vi "界面UI.vi"() -> ()   [LabVIEW 2016, in "德润超标留样.lvlib"]
uses:
  <vilib>/Utility/miscctls.llb/LVPointTypeDef.ctl
panel:
  out "超标留样运行状态":T1(xcontrol)
  in  "外控留样设置":bool
  in  "外控留样读取":bool
  in  "串口重开":bool
  in  "读取选择":string(combo)
  in  "超标留样设置":bool
  in  "超标留样读取":bool
  in  "VISA resource name":refnum<visa-resource-name>="COM10" caption="VISA资源名称"
  in  "写入缓冲区":string
  in  "采样模式":enum16{"定时留样", "时间等比", "同步留样", "外控留样", "超标留样"}(ring)
  in  "采样启动":bool
  in  "切换停止":bool
  in  "切换运行":bool
  in  "时间校准":bool
  out "仪器状态":T1 {"仪器时间" format="%<%Y/%m/%d %H:%M:%S>T"; "门状态" items=["关闭", "打开"]; "采样模式" items=["定时留样"=1, "时间等比"=2, "同步留样"=3, "外控留样"=4, "超标留样"=5]; "工作进程" items=["停止中"=0, "启动延时"=1, "外置泵延时"=2, "管路润洗"=3, "管存"=4, "留样"=5, "出水管路排空"=6, "采水管路排空"=7, "待机"=13]; "工作状态" items=["停止", "运行", "系统初始化"]}
  out "读取缓冲区":string
  out "source":string
  out "通讯":bool
  # "德润超标留样"
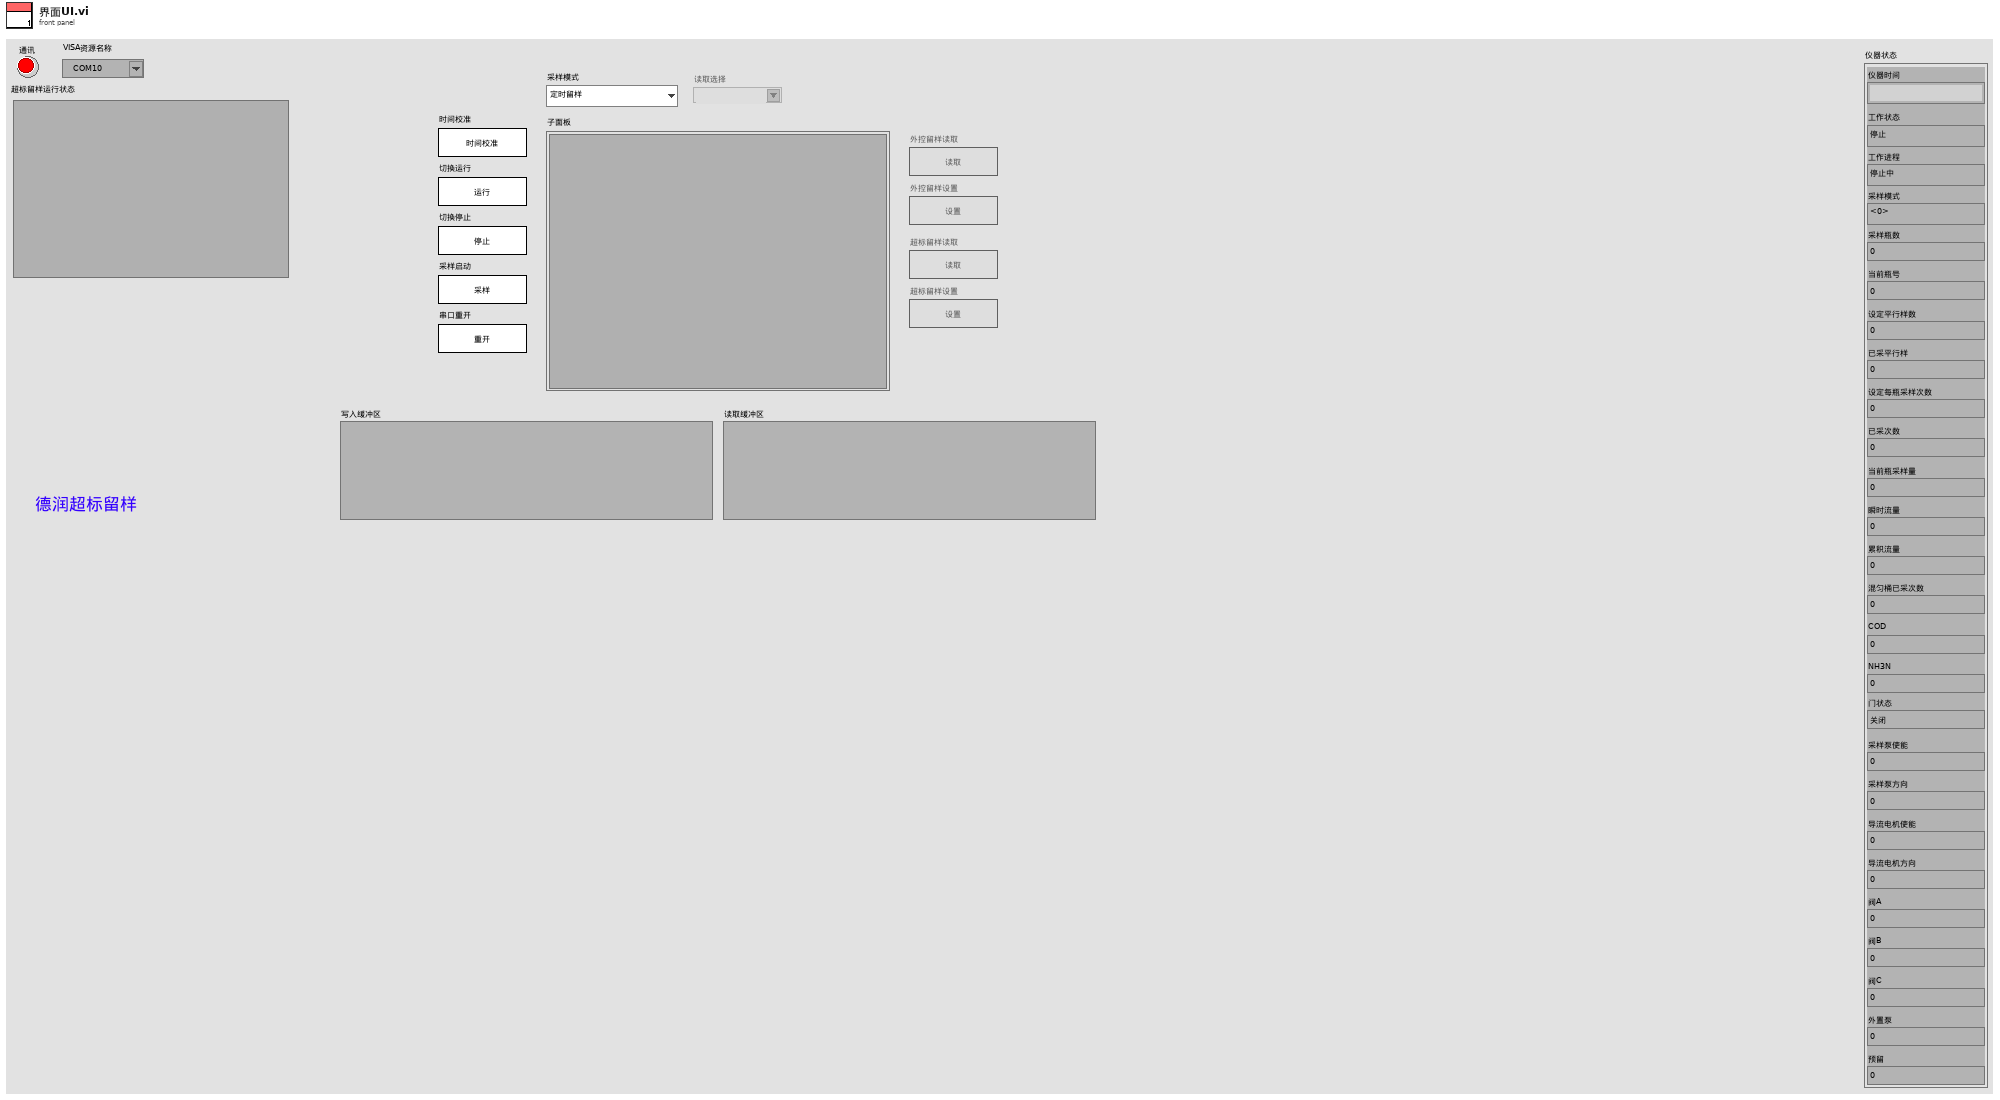
[diagram p1: front panel]
types:
  T1 = cluster{"仪器时间":timestamp, "工作状态":u16, "工作进程":u16, "采样模式":u16, "采样瓶数":dbl, "当前瓶号":dbl, "设定平行样数":dbl, "已采平行样":dbl, "设定每瓶采样次数":dbl, "已采次数":dbl, "当前瓶采样量":dbl, "瞬时流量":dbl, "累积流量":dbl, "混匀桶已采次数":dbl, "COD":dbl, "NH3N":dbl, "门状态":u16, "采样泵使能":dbl, "采样泵方向":dbl, "导流电机使能":dbl, "导流电机方向":dbl, "阀A":dbl, "阀B":dbl, "阀C":dbl, "外置泵":dbl, "预留":dbl}
  T2 = typedef "LVPointTypeDef.ctl" = cluster{"Horizontal":i16, "Vertical":i16}
  T3 = enum32{"Bad", "Idle", "Run top level", "Running"}
  T4 = cluster{"当前瓶号：":dbl, "平行样：":dbl, "留样瓶数：":dbl, "每瓶次数：":dbl, "每次留样：":dbl}
  T5 = cluster{"当前瓶号：":dbl, "平行样：":dbl, "留样瓶数：":dbl, "每瓶次数：":dbl, "每次留样：":dbl, "时间间隔：":dbl, "COD联机：":u16, "氨氮联机：":u16, "4mA浓度：":dbl, "20mA浓度：":dbl, "超标浓度：":dbl, "4mA浓度：":dbl, "20mA浓度:":dbl, "超标浓度：":dbl}
  T6 = enum8{"Enabled", "Disabled", "Disabled and Grayed Out"}
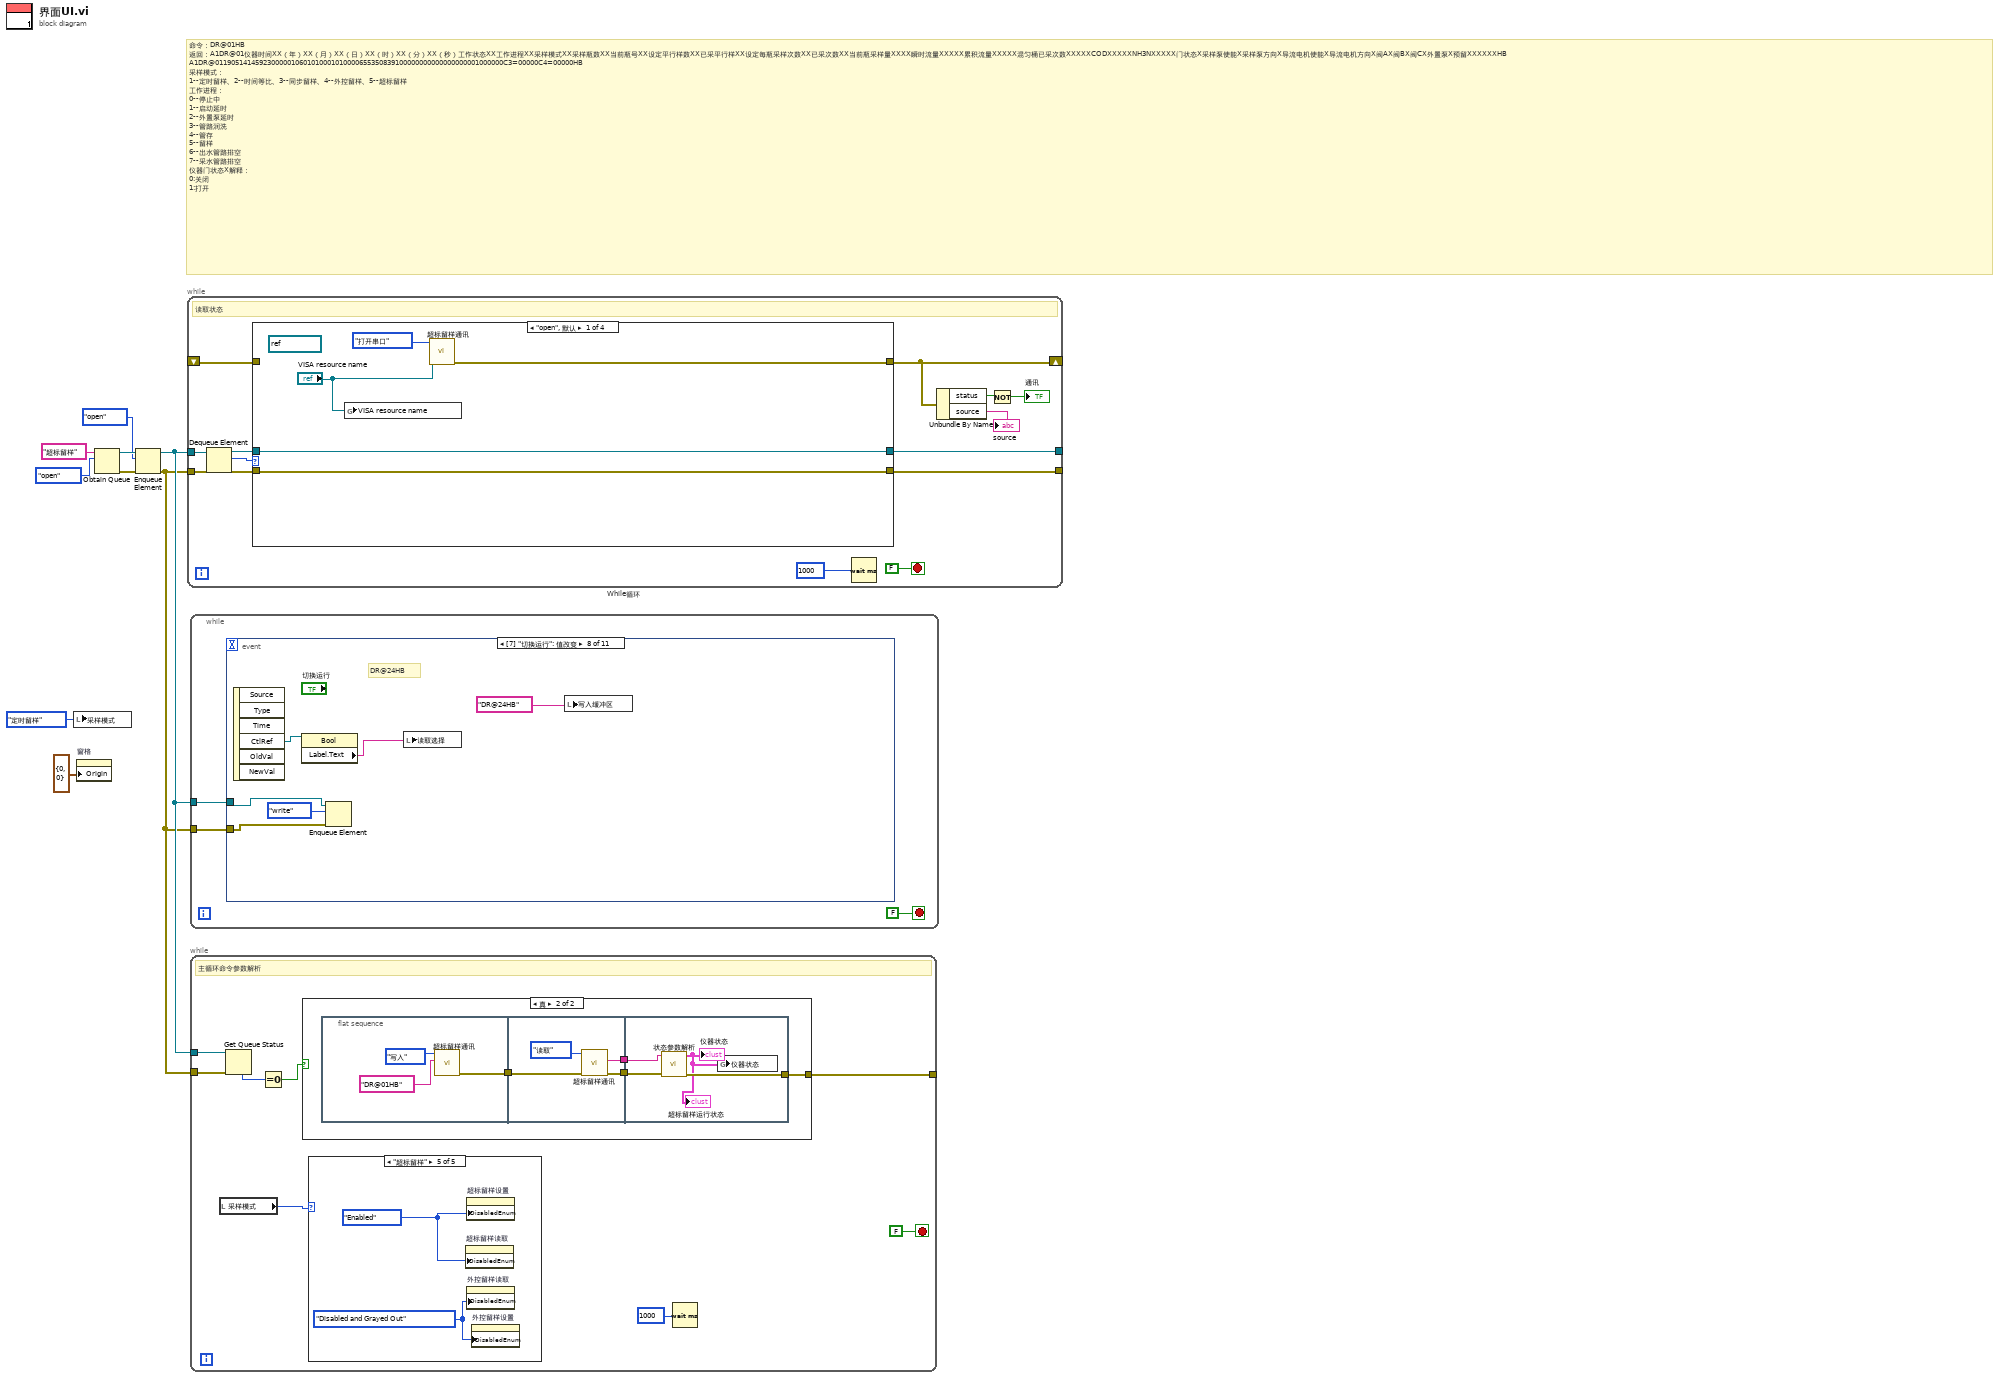
[diagram p0: block diagram]
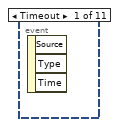
[diagram p2: hidden frame]
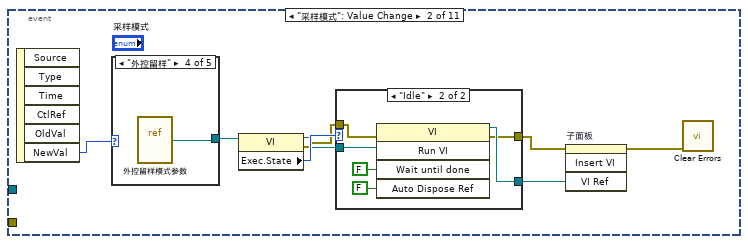
[diagram p3: hidden frame]
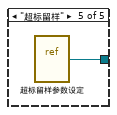
[diagram p8: hidden frame]
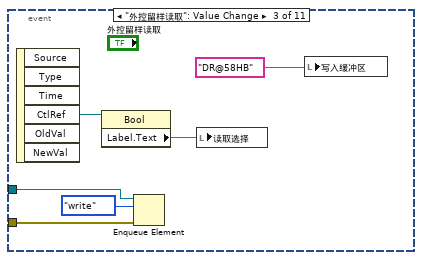
[diagram p9: hidden frame]
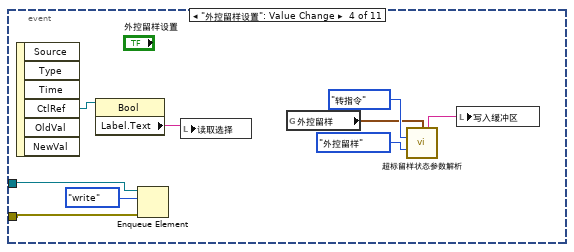
[diagram p10: hidden frame]
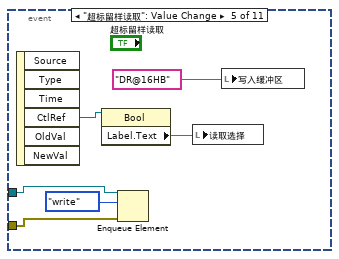
[diagram p11: hidden frame]
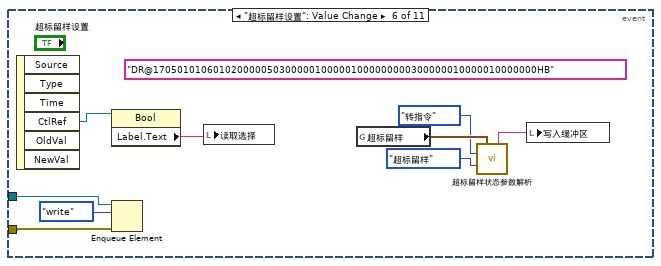
[diagram p12: hidden frame]
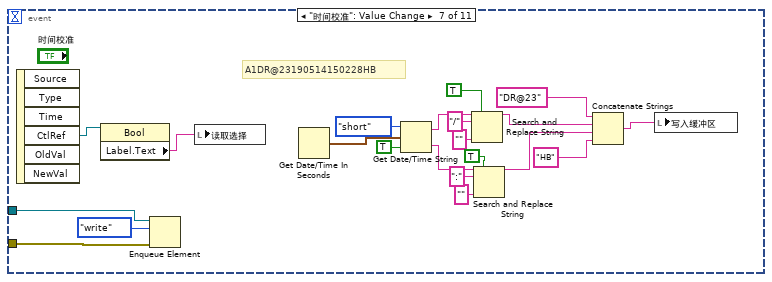
[diagram p13: hidden frame]
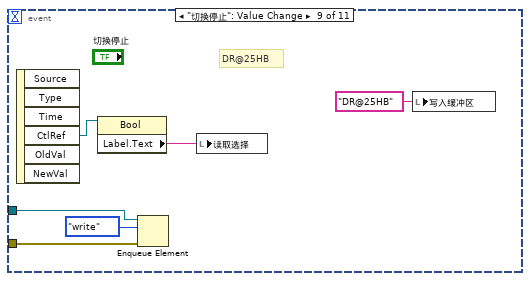
[diagram p14: hidden frame]
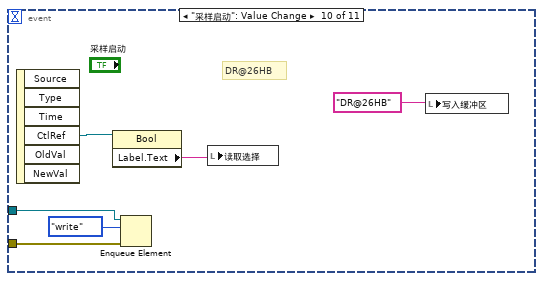
[diagram p15: hidden frame]
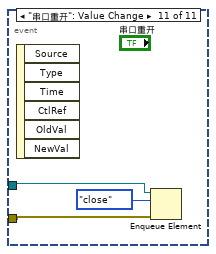
[diagram p16: hidden frame]
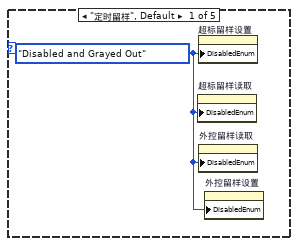
[diagram p18: hidden frame]
diagram:
  # "命令：DR@01HB\n返回：A1DR@01仪器时间XX（年）XX（月）XX（日）XX（时）XX（分）XX（秒）工作状态XX工作进程XX采样模式XX采样瓶数XX当前瓶号XX设定平行样数XX已采平行样XX设定每瓶采样次数XX已采次数XX当前瓶采样量XXXX瞬时流量XXXXX累积流量XXXXX混匀桶已采次数XXXXXCODXXXXXNH3NXXXXX门状态X采样泵使能X采样泵方向X导流电机使能X导流电机方向X阀AX阀BX阀CX外置泵X预留XXXXXXHB\nA1DR@011905141459230000010601010001010000655350839100000000000000000001000000C3=00000C4=00000HB\n采样模式：\n1--定时留样、2--时间等比、3--同步留样、4--外控留样、5--超标留样\n工作进程：\n0--停止中\n1--启动延时\n2--外置泵延时\n3--管路润洗\n4--管存\n5--留样\n6--出水管路排空\n7--采水管路排空\n仪器门状态X解释：\n0:关闭\n1:打开"
  n1 = local write "采样模式"(enum16{"定时留样", "时间等比", "同步留样", "外控留样", "超标留样"}."定时留样" ("采样模式")) -> ()
  n2 = property on="窗格" class="Pane"("Origin"=T2 {"Horizontal"=0, "Vertical"=0} ("原点")) -> ()  [unwired: 2 in, 2 out]
  n3 = Obtain Queue(name (unnamed)="超标留样" ("名称（未命名）"), element data type=enum16{"open", "read", "write", "close"}."open") -> (queue out=w7:refnum<queue>, error out=w6:errorcluster)  [unwired: 3 in, 1 out]
  n4 = Enqueue Element(queue=w7, element=enum16{"open", "read", "write", "close"}."open", error in (no error)=w6) -> (queue out=w3:refnum<queue>, error out=w2:errorcluster)  [unwired: 1 in, 1 out]
  n5 = while "While循环" {
    tunnel: w3 -> [w21]
    tunnel: w2 -> [w20]
    tunnel: [w16] -> _
    tunnel: [w15] -> _
    shift-right: [w10] -> _
    shift-left: _ -> [w14]
    stop <- FALSE stop-if-true
    # "读取状态"
    n6 = Dequeue Element(queue=w21, error in (no error)=w20) -> (queue out=w18:refnum<queue>, element=w19:enum16{"open", "read", "write", "close"}, error out=w17:errorcluster)  [unwired: 1 in, 1 out]
    n7 = case shown="\"open\", 默认" w19 {
      tunnel: [w27 w34 w57 w69] -> w10
      tunnel: w18 -> [w26 w32 w62 w68]
      tunnel: w17 -> [w25 w31 w61 w67]
      tunnel: [w26 w32 w60 w65] -> w16
      tunnel: [w25 w31 w59 w64] -> w15
      tunnel: w14 -> [_ w35 w58 w71]
      frame "open", Default {
        (unwired) refnum<visa-resource-name> "COM2" ("VISA resource name")
        n8 = global write "超标留样全局.vi" "VISA resource name"("VISA resource name") -> ()
        n9 = call "超标留样通讯.vi"("VISA resource name"="VISA resource name", "功能输入"=enum16{"打开串口", "写入", "读取", "关闭串口"}."打开串口") -> ("error out"=w27:errorcluster)  [unwired: 7 in, 2 out]
      }
      frame "read" {
        n10 = call "超标留样通讯.vi"("error in (no error)"=w35, "功能输入"=enum16{"打开串口", "写入", "读取", "关闭串口"}."读取") -> ("error out"=w34:errorcluster, "读取缓冲区"=w29:string)  [unwired: 7 in, 1 out]
        "读取缓冲区" <- w29
        n11 = case shown="\"外控留样读取\"" "读取选择" {
          tunnel: w29 -> [w36 w43 w54]
          frame "超标留样读取" {
            n12 = flat-sequence {
              tunnel: w36 -> [w39]
              frame #0 {
                n13 = call "超标留样状态参数解析.vi"("输入字符串"=w39, "解析/转指令"=enum16{"解析", "转指令"}."解析", "模式选择"=enum16{"外控留样", "超标留样"}."超标留样") -> ()  [unwired: 11 in, 2 out]
              }
              frame #1 {
                n14 = global write "超标留样全局.vi" "读取更新"(TRUE ("读取更新")) -> ()
              }
              frame #2 {
                n15 = Wait (ms)(milliseconds to wait=u32 500 ("等待时间（毫秒）")) -> ()  [unwired: 1 out]
              }
              frame #3 {
                n16 = global write "超标留样全局.vi" "读取更新"(FALSE ("读取更新")) -> ()
              }
            }
          }
          frame "外控留样读取" {
            n17 = flat-sequence {
              tunnel: w43 -> [w44]
              frame #0 {
                n18 = call "超标留样状态参数解析.vi"("输入字符串"=w44, "解析/转指令"=enum16{"解析", "转指令"}."解析", "模式选择"=enum16{"外控留样", "超标留样"}."外控留样") -> ()  [unwired: 11 in, 2 out]
              }
              frame #1 {
                n19 = global write "超标留样全局.vi" "外控留样读取更新"(TRUE ("读取更新")) -> ()
              }
              frame #2 {
                n20 = Wait (ms)(milliseconds to wait=u32 500 ("等待时间（毫秒）")) -> ()  [unwired: 1 out]
              }
              frame #3 {
                n21 = global write "超标留样全局.vi" "外控留样读取更新"(FALSE ("读取更新")) -> ()
              }
            }
          }
          frame "超标留样设置", Default {
            n22 = String Subset(string=w54, offset (0)=5 ("偏移量(0)")) -> (substring=w52:string)  [unwired: 1 in]
            n23 = Search/Split String(string=w52, search string/char (-)="HB" ("搜索字符串/字符(-)")) -> (substring before match=w50:string)  [unwired: 1 in, 2 out]
            n24 = One Button Dialog(message=w50) -> ()  [unwired: 1 in, 1 out]
          }
        }
      }
      frame "write" {
        n25 = call "超标留样通讯.vi"("error in (no error)"=w58, "写入缓冲区"="写入缓冲区", "功能输入"=enum16{"打开串口", "写入", "读取", "关闭串口"}."写入") -> ("error out"=w57:errorcluster)  [unwired: 6 in, 2 out]
        n26 = Enqueue Element(queue=w62, element=enum16{"open", "read", "write", "close"}."read" ("元素"), error in (no error)=w61) -> (queue out=w60:refnum<queue>, error out=w59:errorcluster)  [unwired: 1 in, 1 out]
      }
      frame "close" {
        n27 = call "超标留样通讯.vi"("error in (no error)"=w71, "功能输入"=enum16{"打开串口", "写入", "读取", "关闭串口"}."关闭串口") -> ("error out"=w69:errorcluster)  [unwired: 7 in, 2 out]
        n28 = Enqueue Element(queue=w68, element=enum16{"open", "read", "write", "close"}."open" ("元素"), error in (no error)=w67) -> (queue out=w65:refnum<queue>, error out=w64:errorcluster)  [unwired: 1 in, 1 out]
      }
    }
    n29 = Wait (ms)(milliseconds to wait=u32 1000 ("等待时间（毫秒）")) -> ()  [unwired: 1 out]
    n30 = Unbundle By Name(w10) -> ("status"=w11:bool, "source"=→"source":string)
    n31 = Not(x=w11) -> (.not. x?=→"通讯":bool)
  }
  n32 = while {
    tunnel: w3 -> [w73]
    tunnel: w2 -> [w72]
    stop <- FALSE stop-if-true
    n33 = event shown="[7] \"切换运行\": 值改变" {
      selector: _ -> [_ _ _ _ _ _ _ _ _ _ _]
      dyn-events: _ -> [_ _ _ _ _ _ _ _ _ _ _]
      timeout: _ -> [_ _ _ _ _ _ _ _ _ _ _]
      tunnel: w73 -> [_ _ w95 w106 w111 w121 w142 w147 w153 w159 w163]
      tunnel: w72 -> [_ _ w96 w105 w110 w120 w141 w146 w152 w158 w162]
      event Timeout {
        n34 = event-data() -> ()  [unwired: 1 in, 3 out]
      }
      event "采样模式": Value Change {
        n35 = event-data() -> ("NewVal"=w82:enum16{"定时留样", "时间等比", "同步留样", "外控留样", "超标留样"})  [unwired: 1 in, 5 out]
        n36 = case shown="\"外控留样\"" w82 {
          tunnel: [_ _ _ w91 w92] -> w81
          frame "定时留样", Default {
          }
          frame "时间等比" {
          }
          frame "同步留样" {
          }
          frame "外控留样" {
            n37 = vi-ref "外控留样模式参数.vi"() -> (w91:refnum<vi>)
          }
          frame "超标留样" {
            n38 = vi-ref "超标留样参数设定.vi"() -> (w92:refnum<vi>)
          }
        }
        n39 = property class="VI"(reference=w81) -> (reference out=w79:refnum<vi>, error out=w77:errorcluster, "Exec.State"=w80:T3)  [unwired: 1 in]
        n40 = case shown="\"Idle\"" w80 {
          tunnel: w79 -> [w84 w90]
          tunnel: [w84 w87] -> w78
          tunnel: w77 -> [w83 w86]
          tunnel: [w83 w85] -> w76
          frame "Bad", Default {
          }
          frame "Idle" {
            n41 = invoke class="VI" method="Run VI"(reference=w90, error in=w86, "Wait until done"=FALSE ("结束前等待"), "Auto Dispose Ref"=FALSE ("自动销毁引用")) -> (reference out=w87:refnum<vi>, error out=w85:errorcluster)  [unwired: 1 in, 3 out]
          }
        }
        n42 = invoke on="子面板" class="SubPnl" method="Insert VI"(error in=w76, "VI Ref"=w78) -> (error out=w75:errorcluster)  [unwired: 2 in, 3 out]
        n43 = call <vilib>:"Clear Errors.vi"("error in (no error)"=w75) -> ()  [unwired: 5 in, 2 out]
      }
      event "外控留样读取": Value Change {
        n44 = event-data() -> ("CtlRef"=w94:refnum<vi>)  [unwired: 1 in, 5 out]
        n45 = property class="Bool"(reference=w94) -> ("Label.Text"=w93:string)  [unwired: 1 in, 2 out]
        n46 = Enqueue Element(queue=w95, element=enum16{"open", "read", "write", "close"}."write" ("元素"), error in (no error)=w96) -> ()  [unwired: 1 in, 3 out]
        n47 = local write "读取选择"(w93) -> ()
        n48 = local write "写入缓冲区"("DR@58HB") -> ()
      }
      event "外控留样设置": Value Change {
        n49 = event-data() -> ("CtlRef"=w100:refnum<vi>)  [unwired: 1 in, 5 out]
        n50 = property class="Bool"(reference=w100) -> ("Label.Text"=w99:string)  [unwired: 1 in, 2 out]
        n51 = Enqueue Element(queue=w106, element=enum16{"open", "read", "write", "close"}."write" ("元素"), error in (no error)=w105) -> ()  [unwired: 1 in, 3 out]
        n52 = local write "读取选择"(w99) -> ()
        n53 = global read "超标留样全局.vi" "外控留样"() -> (w101:T4)
        n54 = call "超标留样状态参数解析.vi"("外控留样"=w101, "解析/转指令"=enum16{"解析", "转指令"}."转指令", "模式选择"=enum16{"外控留样", "超标留样"}."外控留样") -> ("输出字符串"=w102:string)  [unwired: 11 in, 1 out]
        n55 = local write "写入缓冲区"(w102) -> ()
      }
      event "超标留样读取": Value Change {
        n56 = event-data() -> ("CtlRef"=w109:refnum<vi>)  [unwired: 1 in, 5 out]
        n57 = property class="Bool"(reference=w109) -> ("Label.Text"=w108:string)  [unwired: 1 in, 2 out]
        n58 = Enqueue Element(queue=w111, element=enum16{"open", "read", "write", "close"}."write" ("元素"), error in (no error)=w110) -> ()  [unwired: 1 in, 3 out]
        n59 = local write "读取选择"(w108) -> ()
        n60 = local write "写入缓冲区"("DR@16HB") -> ()
      }
      event "超标留样设置": Value Change {
        (unwired) "DR@1705010106010200000503000001000001000000000300000010000010000000HB"
        n61 = event-data() -> ("CtlRef"=w115:refnum<vi>)  [unwired: 1 in, 5 out]
        n62 = property class="Bool"(reference=w115) -> ("Label.Text"=w114:string)  [unwired: 1 in, 2 out]
        n63 = Enqueue Element(queue=w121, element=enum16{"open", "read", "write", "close"}."write" ("元素"), error in (no error)=w120) -> ()  [unwired: 1 in, 3 out]
        n64 = local write "读取选择"(w114) -> ()
        n65 = global read "超标留样全局.vi" "超标留样"() -> (w119:T5)
        n66 = call "超标留样状态参数解析.vi"("超标留样"=w119, "解析/转指令"=enum16{"解析", "转指令"}."转指令", "模式选择"=enum16{"外控留样", "超标留样"}."超标留样") -> ("输出字符串"=w116:string)  [unwired: 11 in, 1 out]
        n67 = local write "写入缓冲区"(w116) -> ()
      }
      event "时间校准": Value Change {
        # "A1DR@23190514150228HB"
        n68 = event-data() -> ("CtlRef"=w124:refnum<vi>)  [unwired: 1 in, 5 out]
        n69 = property class="Bool"(reference=w124) -> ("Label.Text"=w123:string)  [unwired: 1 in, 2 out]
        n70 = Enqueue Element(queue=w142, element=enum16{"open", "read", "write", "close"}."write" ("元素"), error in (no error)=w141) -> ()  [unwired: 1 in, 3 out]
        n71 = local write "读取选择"(w123) -> ()
        n72 = Get Date/Time In Seconds() -> (seconds since 1Jan1904=w137:timestamp)
        n73 = Get Date/Time String(date format (0)=enum16{"short", "long", "abbreviated"}."short" ("日期格式(0)"), seconds (now)=w137, want seconds? (F)=TRUE ("需要秒？(F)")) -> (date string=w136:string, time string=w129:string)
        n74 = Search and Replace String(replace all?=TRUE ("替换全部？(F)"), input string=w136, search string="/" ("搜索字符串"), replace string="" ("替换字符串(\"\")")) -> (result string=w128:string)  [unwired: 4 in, 3 out]
        n75 = Search and Replace String(replace all?=TRUE ("替换全部？(F)"), input string=w129, search string=":" ("搜索字符串"), replace string="" ("替换字符串(\"\")")) -> (result string=w127:string)  [unwired: 4 in, 3 out]
        n76 = Concatenate Strings("DR@23" ("写入缓冲区"), w128, w127, "HB" ("写入缓冲区")) -> (w125:string)
        n77 = local write "写入缓冲区"(w125) -> ()
      }
      event "切换运行": Value Change {
        # "DR@24HB"
        n78 = event-data() -> ("CtlRef"=w145:refnum<vi>)  [unwired: 1 in, 5 out]
        n79 = property class="Bool"(reference=w145) -> ("Label.Text"=w144:string)  [unwired: 1 in, 2 out]
        n80 = Enqueue Element(queue=w147, element=enum16{"open", "read", "write", "close"}."write" ("元素"), error in (no error)=w146) -> ()  [unwired: 1 in, 3 out]
        n81 = local write "读取选择"(w144) -> ()
        n82 = local write "写入缓冲区"("DR@24HB") -> ()
      }
      event "切换停止": Value Change {
        # "DR@25HB"
        n83 = event-data() -> ("CtlRef"=w151:refnum<vi>)  [unwired: 1 in, 5 out]
        n84 = property class="Bool"(reference=w151) -> ("Label.Text"=w150:string)  [unwired: 1 in, 2 out]
        n85 = Enqueue Element(queue=w153, element=enum16{"open", "read", "write", "close"}."write" ("元素"), error in (no error)=w152) -> ()  [unwired: 1 in, 3 out]
        n86 = local write "读取选择"(w150) -> ()
        n87 = local write "写入缓冲区"("DR@25HB" ("写入缓冲区")) -> ()
      }
      event "采样启动": Value Change {
        # "DR@26HB"
        n88 = event-data() -> ("CtlRef"=w157:refnum<vi>)  [unwired: 1 in, 5 out]
        n89 = property class="Bool"(reference=w157) -> ("Label.Text"=w156:string)  [unwired: 1 in, 2 out]
        n90 = Enqueue Element(queue=w159, element=enum16{"open", "read", "write", "close"}."write" ("元素"), error in (no error)=w158) -> ()  [unwired: 1 in, 3 out]
        n91 = local write "读取选择"(w156) -> ()
        n92 = local write "写入缓冲区"("DR@26HB") -> ()
      }
      event "串口重开": Value Change {
        n93 = event-data() -> ()  [unwired: 1 in, 6 out]
        n94 = Enqueue Element(queue=w163, element=enum16{"open", "read", "write", "close"}."close" ("元素"), error in (no error)=w162) -> ()  [unwired: 1 in, 3 out]
      }
    }
  }
  n95 = while {
    tunnel: [w170] -> _
    tunnel: w3 -> [w168]
    tunnel: w2 -> [w167]
    stop <- FALSE stop-if-true
    # "主循环命令参数解析"
    n96 = local read "采样模式"() -> (w169:enum16{"定时留样", "时间等比", "同步留样", "外控留样", "超标留样"})
    n97 = Get Queue Status(queue=w168, error in (no error)=w167) -> (# elements in queue=w166:i32)  [unwired: 1 in, 7 out]
    n98 = Equal To 0?(x=w166) -> (x = 0?=w165:bool)
    n99 = case shown="真" w165 {
      tunnel: [_ w173] -> w170
      frame False {
      }
      frame True {
        n100 = flat-sequence {
          tunnel: [w177] -> w176
          tunnel: w176 -> [w182]
          tunnel: [w181] -> w175
          tunnel: [w180] -> w174
          tunnel: w175 -> [w187]
          tunnel: w174 -> [w186]
          tunnel: [w185] -> w173
          frame #0 {
            n101 = call "超标留样通讯.vi"("写入缓冲区"="DR@01HB", "功能输入"=enum16{"打开串口", "写入", "读取", "关闭串口"}."写入") -> ("error out"=w177:errorcluster)  [unwired: 7 in, 2 out]
          }
          frame #1 {
            n102 = call "超标留样通讯.vi"("error in (no error)"=w182, "功能输入"=enum16{"打开串口", "写入", "读取", "关闭串口"}."读取") -> ("error out"=w181:errorcluster, "读取缓冲区"=w180:string)  [unwired: 7 in, 1 out]
          }
          frame #2 {
            n103 = call "状态参数解析.vi"("error in (no error)"=w187, "字符串"=w186) -> ("error out"=w185:errorcluster, "簇"=w184:T1)  [unwired: 8 in]
            "仪器状态" <- w184
            "超标留样运行状态" <- w184
            n104 = global write "超标留样全局.vi" "仪器状态"(w184) -> ()
          }
        }
      }
    }
    n105 = case shown="\"超标留样\"" w169 {
      frame "定时留样", Default {
        w188 = T6."Disabled and Grayed Out" ("禁用")
        n106 = property on="超标留样读取" class="Bool"("DisabledEnum"=w188) -> ()  [unwired: 2 in, 2 out]
        n107 = property on="超标留样设置" class="Bool"("DisabledEnum"=w188) -> ()  [unwired: 2 in, 2 out]
        n108 = property on="外控留样读取" class="Bool"("DisabledEnum"=w188) -> ()  [unwired: 2 in, 2 out]
        n109 = property on="外控留样设置" class="Bool"("DisabledEnum"=w188) -> ()  [unwired: 2 in, 2 out]
      }
      frame "时间等比" {
      }
      frame "同步留样" {
      }
      frame "外控留样" {
        w189 = T6."Enabled" ("禁用")
        w190 = T6."Disabled and Grayed Out" ("禁用")
        n110 = property on="超标留样读取" class="Bool"("DisabledEnum"=w190) -> ()  [unwired: 2 in, 2 out]
        n111 = property on="超标留样设置" class="Bool"("DisabledEnum"=w190) -> ()  [unwired: 2 in, 2 out]
        n112 = property on="外控留样读取" class="Bool"("DisabledEnum"=w189) -> ()  [unwired: 2 in, 2 out]
        n113 = property on="外控留样设置" class="Bool"("DisabledEnum"=w189) -> ()  [unwired: 2 in, 2 out]
      }
      frame "超标留样" {
        w191 = T6."Enabled" ("禁用")
        w192 = T6."Disabled and Grayed Out" ("禁用")
        n114 = property on="超标留样读取" class="Bool"("DisabledEnum"=w191) -> ()  [unwired: 2 in, 2 out]
        n115 = property on="超标留样设置" class="Bool"("DisabledEnum"=w191) -> ()  [unwired: 2 in, 2 out]
        n116 = property on="外控留样读取" class="Bool"("DisabledEnum"=w192) -> ()  [unwired: 2 in, 2 out]
        n117 = property on="外控留样设置" class="Bool"("DisabledEnum"=w192) -> ()  [unwired: 2 in, 2 out]
      }
    }
    n118 = Wait (ms)(milliseconds to wait=u32 1000 ("等待时间（毫秒）")) -> ()  [unwired: 1 out]
  }
